vi "matlab_TI2_moveZ.vi"(8 "error in":errorcluster, 10 "dz":dbl) -> (0 "error out":errorcluster, 2 "XYZpos":cluster{dbl, dbl, dbl})   [LabVIEW 2018]
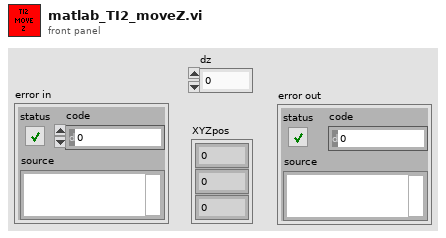
[diagram p1: front panel]
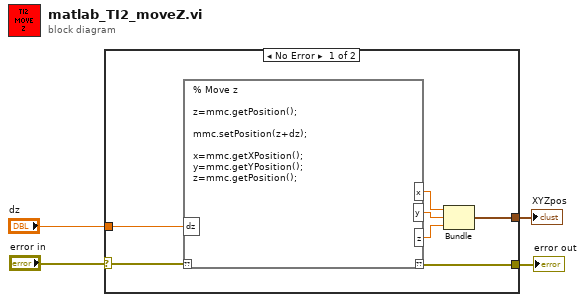
[diagram p0: block diagram]
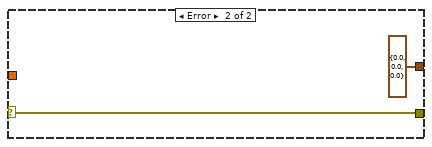
[diagram p2: hidden frame]
diagram:
  n1 = case shown="No Error" "error in" {
    selector: "error in" -> [w11 w13]
    tunnel: [w10 w13] -> w3
    tunnel: "dz" -> [w9 _]
    tunnel: [w5 cluster{dbl, dbl, dbl} {0.0, 0.0, 0.0}] -> w1
    frame No Error {
      n2 = script code="% Move z\n\nz=mmc.getPosition();\n\nmmc.setPosition(z+dz);\n\nx=mmc.getXPosition();\ny=mmc.getYPosition();\nz=mmc.getPosition();"("??"=w11, "dz"=w9) -> ("??"=w10:errorcluster, "x"=w8:dbl, "y"=w7:dbl, "z"=w6:dbl)
      n3 = Bundle(w8, w7, w6) -> (w5:cluster{dbl, dbl, dbl})  [unwired: 1 in]
    }
    frame Error {
    }
  }
  "error out" <- w3
  "XYZpos" <- w1
